vi "Global.vi"() -> ()   [LabVIEW 2014]
panel:
  in  "Enter Filename:":string="Swissknife"
  in  "Visa Sessions":T1={"Parameter Analyzer"="Parameter Analyzer VISA", "Switching Matrix"="Switching Matrix VISA", "Stress Control"="Stress Control VISA", "Switches and Mirrors"="Relay Switches VISA", "XYZ Stage"="XYZ Stage VISA"}
  # "LICENSED MATERIALS – PROPERTY OF IBM\nCopyright IBM Corp. 2016,\nALL RIGHTS RESERVED"
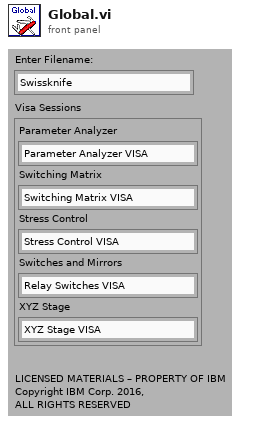
[diagram p1: front panel]
types:
  T1 = cluster{"Parameter Analyzer":string, "Switching Matrix":string, "Stress Control":string, "Switches and Mirrors":string, "XYZ Stage":string}
diagram:
